vi "CheckIfPlayerLost.vi"(9 "StorageSizeExceeded?":bool, 10 "TimedOut?":bool, 11 "HitWall?":bool) -> (2 "Reason":string, 3 "Lost?":bool)   [LabVIEW 2015, in "TronviewGame.lvlib" / "Game.lvclass"]
uses:
  Game.lvclass
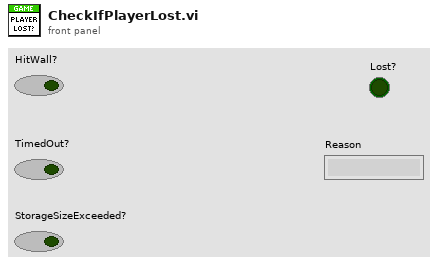
[diagram p1: front panel]
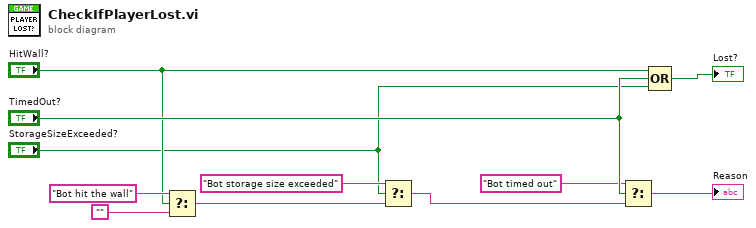
[diagram p0: block diagram]
diagram:
  n1 = Select(t="Bot hit the wall", s="HitWall?", f="") -> (s? t:f=w3:string)
  n2 = Select(t="Bot storage size exceeded", s="StorageSizeExceeded?", f=w3) -> (s? t:f=w2:string)
  n3 = Select(t="Bot timed out", s="TimedOut?", f=w2) -> (s? t:f=→"Reason":string)
  n4 = Compound Arithmetic op=OR("HitWall?", "TimedOut?", "StorageSizeExceeded?") -> (→"Lost?":bool)
